vi "Database.Global.vi"() -> ()   [LabVIEW 2016]
uses:
  Handler/Database.Handler.Data.Status.ctl
  Database.Data.Sets.ctl
panel:
  in  "SetsTab":enum32{"DB"}(tab)
  in  "DB.Sets":T1
  in  "VariantsInUse":string[](array[string])
  out "DB.Status":T2
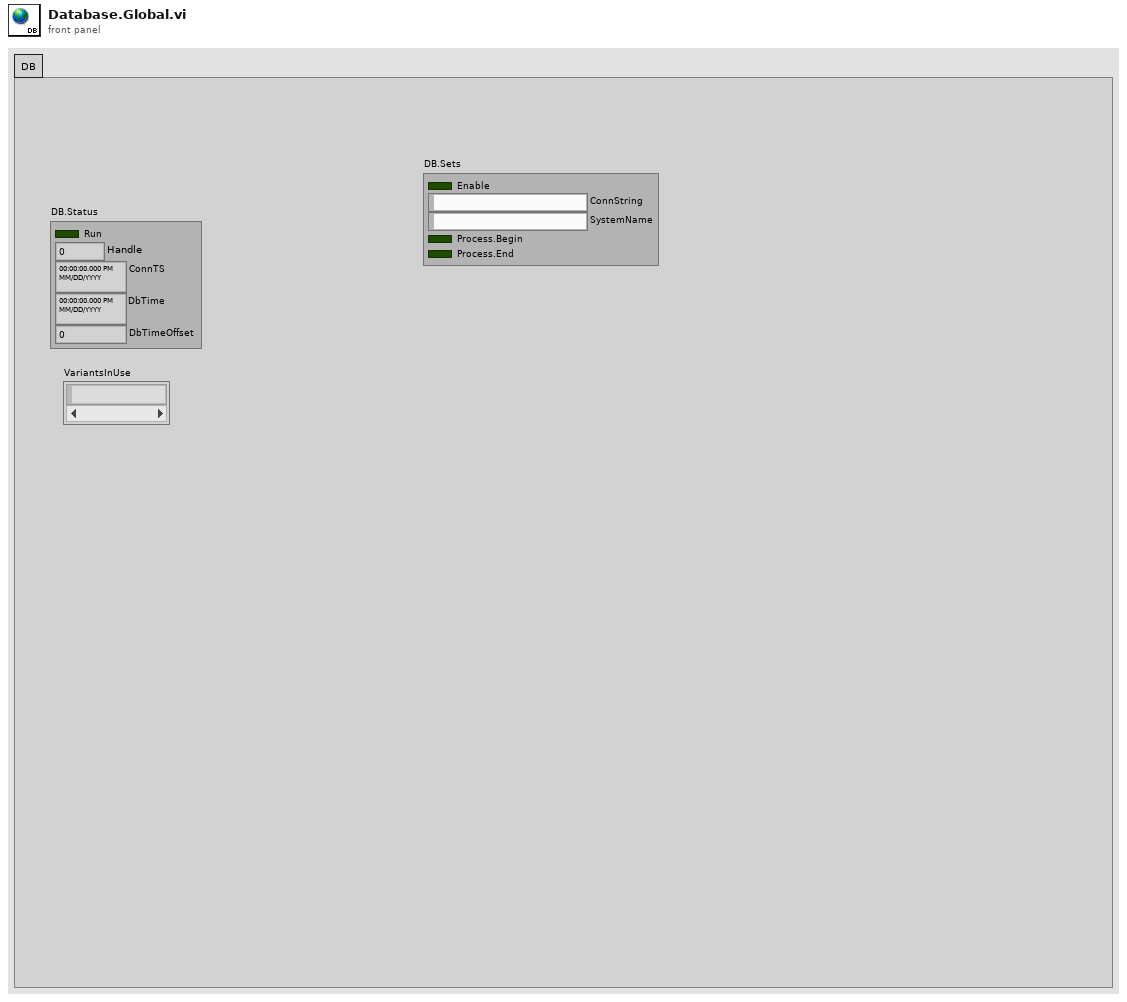
[diagram p1: front panel]
types:
  T1 = typedef "Database.Data.Sets.ctl" = cluster{"Enable":bool, "ConnString":string, "SystemName":string, "Process.Begin":bool, "Process.End":bool}
  T2 = typedef "Database.Handler.Data.Status.ctl" = cluster{"Run":bool, "Handle":i32, "ConnTS":timestamp, "DbTime":timestamp, "DbTimeOffset":dbl}
diagram:
